vi "Update List Log.vi"(9 "Command to Input":string, 11 "reference":refnum<vi>) -> ()   [LabVIEW 2020]
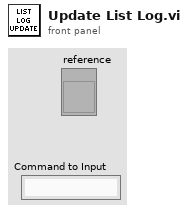
[diagram p1: front panel]
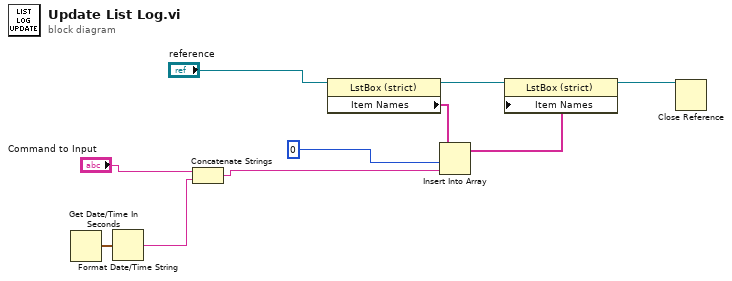
[diagram p0: block diagram]
diagram:
  n1 = Get Date/Time In Seconds() -> (seconds since 1Jan1904=w4:timestamp)
  n2 = Format Date/Time String(seconds (now)=w4) -> (date/time string=w3:string)  [unwired: 2 in]
  n3 = Concatenate Strings("Command to Input", w3) -> (w2:string)
  n4 = property class="LstBox (strict)"(reference="reference") -> (reference out=w7:refnum<vi>, "Item Names"=w10:string[])  [unwired: 1 in, 1 out]
  n5 = Insert Into Array(array=w10, index=0, new element=w2) -> (w9:string[])
  n6 = property class="LstBox (strict)"(reference=w7, "Item Names"=w9) -> (reference out=w6:refnum<vi>)  [unwired: 1 in, 1 out]
  n7 = Close Reference(reference=w6) -> ()  [unwired: 1 in, 1 out]
